vi "data-to-matlab.vi"(8 "error in (no error)":errorcluster, 11 "Config":T1={"Hardware Configuration"={"DAQmx Channel 1"="", "DAQmx Channel 2"="", "DAQmx Channel 3"="", "Channel 1 Name"="", "Channel 2 Name"="", "Channel 3 Name"="", "Input Config Channel 1"=-1, "Input Config Channel 2"=-1, "Input Config Channel 3"=-1, "Offset Channel 1"=0.0, "Offset Channel 2"=0.0, "Offset Channel 3"=0.0, "Scale Channel 1"=0.0, "Scale Channel 2"=0.0, "Scale Channel 3"=0.0, "Sample time"=0, "Samples per second"=0.0, "Sample mode"=0, "Samples per channel"=0, "DAQmx AI Task"="", "DAQmx Channel 4"="", "Channel 3 Name 2"="", "Input Config Channel 4"=-1, "Offset Channel 4"=0.0, "Scale Channel 4"=0.0}, "Logging Configuration"={"Log File Base Path"=path "", "TDMS File Reference"=refnum}} {"Hardware Configuration"."Input Config Channel 4" items=["Default"=-1, "RSE"=10083, "NRSE"=10078, "Differential"=10106, "Pseudodifferential"=12529]; "Hardware Configuration"."Input Config Channel 3" items=["Default"=-1, "RSE"=10083, "NRSE"=10078, "Differential"=10106, "Pseudodifferential"=12529]; "Hardware Configuration"."Input Config Channel 2" items=["Default"=-1, "RSE"=10083, "NRSE"=10078, "Differential"=10106, "Pseudodifferential"=12529]; "Hardware Configuration"."Input Config Channel 1" items=["Default"=-1, "RSE"=10083, "NRSE"=10078, "Differential"=10106, "Pseudodifferential"=12529]; "Hardware Configuration"."Sample mode" items=["Hardware Timed Single Point"=12522, "Finite Samples"=10178, "Continuous Samples"=10123]}) -> (0 "error out":errorcluster)   [LabVIEW 2018]
uses:
  Settings/Settings.ctl
  Acquisition/Hardware Configuration.ctl
  Logging Configuration.ctl
  <vilib>/Waveform/WDTOps.llb/WDT Index Channel DBL.vi
  <vilib>/Waveform/WDTOps.llb/WDT Get Waveform Time Array DBL.vi
  Acquisition/Acquisition.lvlib
  Logging.lvlib
  Settings/Settings.lvlib
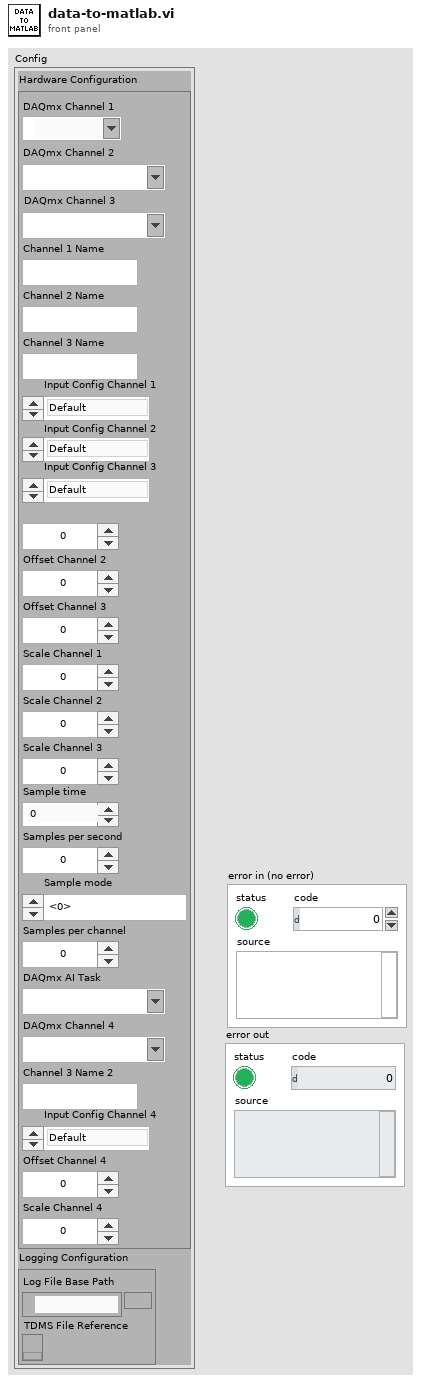
[diagram p1: front panel]
types:
  T1 = typedef "Settings.lvlib/Settings.ctl" = cluster{"Hardware Configuration":T2, "Logging Configuration":T3}
  T2 = typedef "Acquisition.lvlib/Hardware Configuration.ctl" = cluster{"DAQmx Channel 1":tag, "DAQmx Channel 2":tag, "DAQmx Channel 3":tag, "Channel 1 Name":string, "Channel 2 Name":string, "Channel 3 Name":string, "Input Config Channel 1":i32, "Input Config Channel 2":i32, "Input Config Channel 3":i32, "Offset Channel 1":dbl, "Offset Channel 2":dbl, "Offset Channel 3":dbl, "Scale Channel 1":dbl, "Scale Channel 2":dbl, "Scale Channel 3":dbl, "Sample time":u32, "Samples per second":dbl, "Sample mode":u16, "Samples per channel":i32, "DAQmx AI Task":refnum<k21>, "DAQmx Channel 4":tag, "Channel 3 Name 2":string, "Input Config Channel 4":i32, "Offset Channel 4":dbl, "Scale Channel 4":dbl}
  T3 = typedef "Logging.lvlib/Logging Configuration.ctl" = cluster{"Log File Base Path":path, "TDMS File Reference":refnum<k34>}
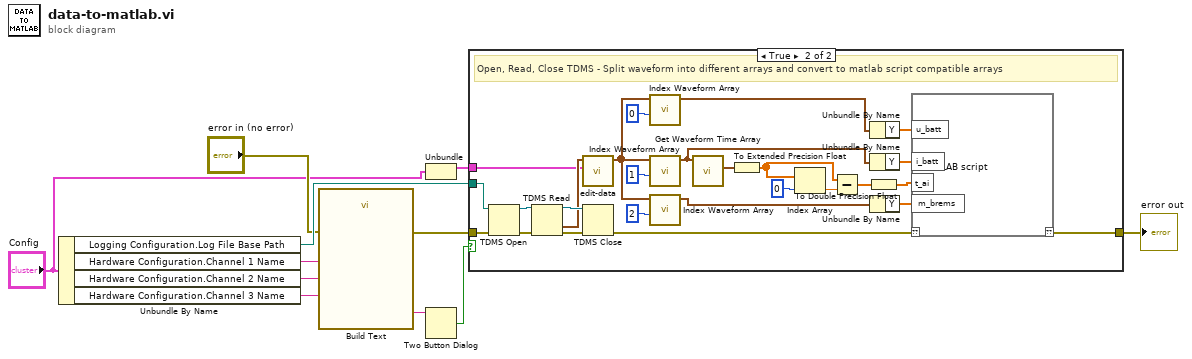
[diagram p0: block diagram]
diagram:
  n1 = Unbundle By Name("Config") -> ("Logging Configuration.Log File Base Path"=w9:path, "Hardware Configuration.Channel 1 Name"=w5:string, "Hardware Configuration.Channel 2 Name"=w6:string, "Hardware Configuration.Channel 3 Name"=w7:string)
  n2 = call "Build Text"("channel1"=w5, "channel2"=w6, "channel3"=w7, "error in (no error)"="error in (no error)") -> ("Result"=w4:string, "error out"=w11:errorcluster)  [unwired: 10 in]
  n3 = Unbundle("Config") -> ("Hardware Configuration"=w1:T2)  [unwired: 1 out]
  n4 = Two Button Dialog(message=w4) -> (T button?=w3:bool)  [unwired: 2 in]
  n5 = case shown="True" w3 {
    tunnel: w9 -> [_ w19]
    tunnel: [w12 w14] -> w10
    tunnel: w11 -> [w12 w18]
    tunnel: w1 -> [_ w16]
    frame False {
      # "If canceled, do nothing"
    }
    frame True {
      # "Open, Read, Close TDMS - Split waveform into different arrays and convert to matlab script compatible arrays"
      n6 = TDMS Open(8:w18, 11:w19) -> (0:w26:errorcluster, 3:w24:refnum<k34>)  [unwired: 5 in]
      n7 = TDMS Read(0:w24, 11:w26) -> (4:w25:refnum<k34>, 10:w17:waveform(dbl)[], 15:w27:errorcluster)  [unwired: 6 in, 3 out]
      n8 = call "edit-data.vi"("Hardware Resources in"=w16, "data"=w17) -> ("Array of Waveform"=w13:waveform(dbl)[])  [unwired: 9 in]
      n9 = TDMS Close(8:w27, 11:w25) -> (0:w15:errorcluster)  [unwired: 1 out]
      n10 = call-poly <vilib>:"Index Waveform Array.vi"("index"=0, "waveform array"=w13) -> ("waveform"=w29:waveform(dbl))  [unwired: 8 in, 1 out]
      n11 = call-poly <vilib>:"Index Waveform Array.vi"("index"=1, "waveform array"=w13) -> ("waveform"=w28:waveform(dbl))  [unwired: 8 in, 1 out]
      n12 = call-poly <vilib>:"Index Waveform Array.vi"("index"=2, "waveform array"=w13) -> ("waveform"=w35:waveform(dbl))  [unwired: 8 in, 1 out]
      n13 = call-poly <vilib>:"Get Waveform Time Array.vi"("waveform in"=w28) -> ("X array"=w31:timestamp[])  [unwired: 9 in, 1 out]
      n14 = To Extended Precision Float(1:w31) -> (0:w32:ext[])
      n15 = Index Array(array=w32, index=0) -> (element=w33:ext)
      n16 = Subtract(x=w32, y=w33) -> (x-y=w37:ext[])
      n17 = To Double Precision Float(number=w37) -> (double precision float=w38:dbl[])
      n18 = Unbundle By Name(w29) -> ("Y"=w34:dbl[])
      n19 = Unbundle By Name(w28) -> ("Y"=w30:dbl[])
      n20 = Unbundle By Name(w35) -> ("Y"=w36:dbl[])
      n21 = script code="MATLAB script"("??"=w15, "i_batt"=w30, "t_ai"=w38, "u_batt"=w34, "m_brems"=w36) -> ("??"=w14:errorcluster)
    }
  }
  "error out" <- w10
